vi "New from string.vi"(11 "String":string) -> (3 "output cluster":refnum<class "MsgPackString.lvclass">)   [LabVIEW 2020, in "MessagePack.lvlib" / "MsgPackString.lvclass"]
uses:
  MsgPackString.lvclass
  MsgPackString.lvclass/MsgPackString.ctl
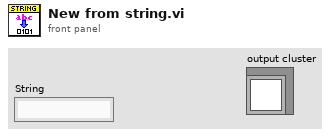
[diagram p1: front panel]
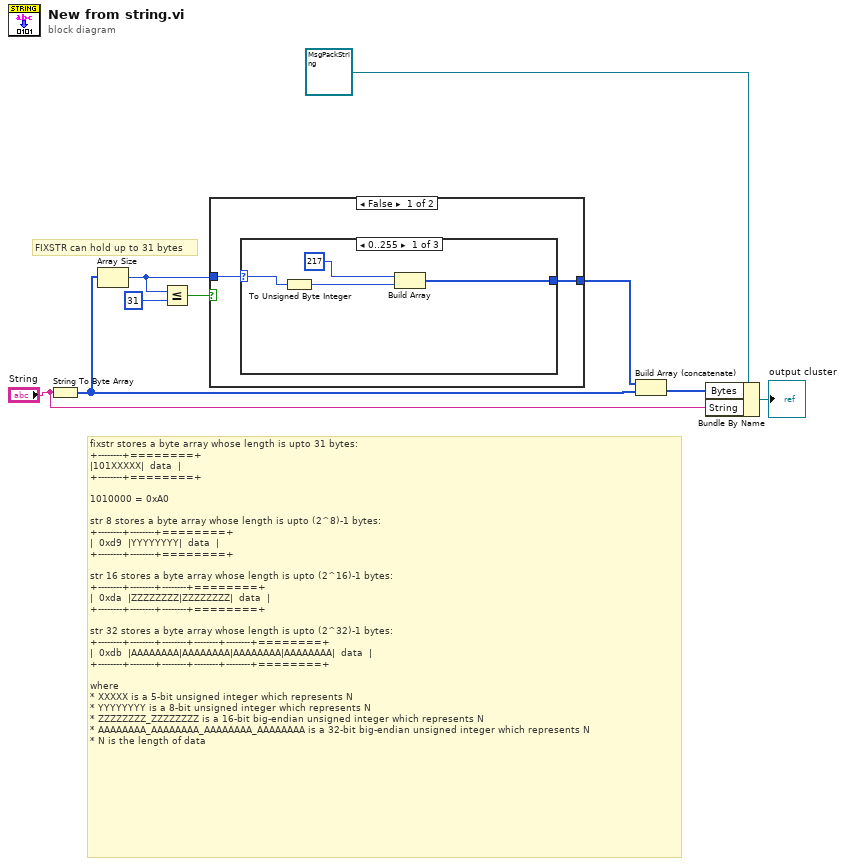
[diagram p0: block diagram]
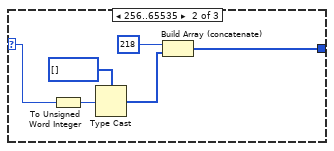
[diagram p2: hidden frame]
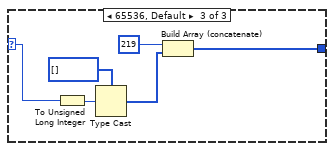
[diagram p3: hidden frame]
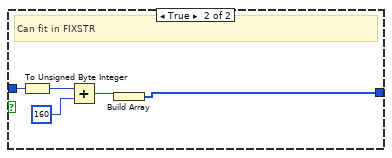
[diagram p4: hidden frame]
diagram:
  # "fixstr stores a byte array whose length is upto 31 bytes:\n+--------+========+\n|101XXXXX|  data  |\n+--------+========+\n\n1010000 = 0xA0\n\nstr 8 stores a byte array whose length is upto (2^8)-1 bytes:\n+--------+--------+========+\n|  0xd9  |YYYYYYYY|  data  |\n+--------+--------+========+\n\nstr 16 stores a byte array whose length is upto (2^16)-1 bytes:\n+--------+--------+--------+========+\n|  0xda  |ZZZZZZZZ|ZZZZZZZZ|  data  |\n+--------+--------+--------+========+\n\nstr 32 stores a byte array whose length is upto (2^32)-1 bytes:\n+--------+--------+--------+--------+--------+========+\n|  0xdb  |AAAAAAAA|AAAAAAAA|AAAAAAAA|AAAAAAAA|  data  |\n+--------+--------+--------+--------+--------+========+\n\nwhere\n* XXXXX is a 5-bit unsigned integer which represents N\n* YYYYYYYY is a 8-bit unsigned integer which represents N\n* ZZZZZZZZ_ZZZZZZZZ is a 16-bit big-endian unsigned integer which represents N\n* AAAAAAAA_AAAAAAAA_AAAAAAAA_AAAAAAAA is a 32-bit big-endian unsigned integer which represents N\n* N is the length of data"
  # "FIXSTR can hold up to 31 bytes"
  n1 = String To Byte Array(string="String") -> (unsigned byte array=w7:u8[])
  n2 = Array Size(array=w7) -> (size(s)=w6:i32)
  n3 = Less Or Equal?(x=w6, y=31) -> (x <= y?=w8:bool)
  n4 = case shown="False" w8 {
    tunnel: w6 -> [w11 w32]
    tunnel: [w10 w28] -> w5
    frame False {
      n5 = case shown="0..255" w11 {
        selector: w11 -> [w15 w19 w22]
        tunnel: [w12 w20 w26] -> w10
        frame 0..255 {
          n6 = To Unsigned Byte Integer(number=w15) -> (unsigned 8bit integer=w13:u8)
          n7 = Build Array(u8 217 ("y"), w13) -> (w12:u8[])
        }
        frame 256..65535 {
          n8 = To Unsigned Word Integer(number=w19) -> (unsigned 16bit integer=w17:u16)
          n9 = Type Cast(type=u8[] [] ("bytes"), x=w17) -> (*(type *) &x=w16:u8[])
          n10 = Build Array (concatenate)(u8 218 ("y"), w16) -> (w20:u8[])
        }
        frame 65536, Default {
          n11 = To Unsigned Long Integer(number=w22) -> (unsigned 32bit integer=w23:u32)
          n12 = Type Cast(type=u8[] [] ("bytes"), x=w23) -> (*(type *) &x=w24:u8[])
          n13 = Build Array (concatenate)(u8 219 ("y"), w24) -> (w26:u8[])
        }
      }
    }
    frame True {
      # "Can fit in FIXSTR"
      n14 = To Unsigned Byte Integer(number=w32) -> (unsigned 8bit integer=w31:u8)
      n15 = Add(x=w31, y=u8 160) -> (x+y=w29:u8)
      n16 = Build Array(w29) -> (w28:u8[])
    }
  }
  n17 = Build Array (concatenate)(w5, w7) -> (w2:u8[])
  n18 = Bundle By Name(cluster=refnum<class "MsgPackString.lvclass"> refnum ("MessagePack.lvlib:MsgPackString.lvclass"), "Bytes"=w2, "String"="String") -> (→"output cluster":refnum<class "MsgPackString.lvclass">)
